vi "4x 5wire xVDTs.vi"() -> ()   [LabVIEW 2010]
uses:
  <vilib>/Platform/TimedLoop/XDataNode/XDataNode.xnode
  <vilib>/Platform/TimedLoop/XDataNode/timing_clust.ctl
  <vilib>/Platform/TimedLoop/XDataNode/nitl_modes.ctl
  <vilib>/Platform/TimedLoop/XDataNode/wakeup.ctl
  <vilib>/Platform/TimedLoop/XDataNode/XDNodeRunTimeDep.lvlib
  <vilib>/NI Veristand/FPGA/NI_VS FPGA Support.lvlib
  <userlib>/_NI VeriStand FPGA Support/NI VeriStand FPGA Clock Support/NI_VS FPGA Clock Support.lvlib
panel:
  in  "xVDT3.ScaleFactor1":i32
  in  "xVDT2.ScaleFactor2":i32
  in  "xVDT1.ScaleFactor1":i32
  in  "xVDT3.ScaleFactor2":i32
  in  "xVDT3.Scale2":fxp<+/-,19,5>
  in  "xVDT3.Scale1":fxp<+/-,19,5>
  in  "xVDT2.ScaleFactor1":i32
  in  "xVDT2.Scale2":fxp<+/-,19,5>
  in  "xVDT2.Scale1":fxp<+/-,19,5>
  in  "xVDT1.ScaleFactor2":i32
  in  "xVDT1.Scale2":fxp<+/-,19,5>
  in  "xVDT1.Scale1":fxp<+/-,19,5>
  in  "xVDT0.ScaleFactor1":i32
  in  "xVDT0.ScaleFactor2":i32
  in  "xVDT0.Scale2":fxp<+/-,19,5>
  in  "xVDT0.Scale1":fxp<+/-,19,5>
  in  "Generate IRQ":bool
  in  "Use External Timing":bool
  in  "Write to  RTSI":bool
  in  "Loop Rate (usec)":u32
  in  "Start":bool
  # "5 Wire"
  # "Configuration"
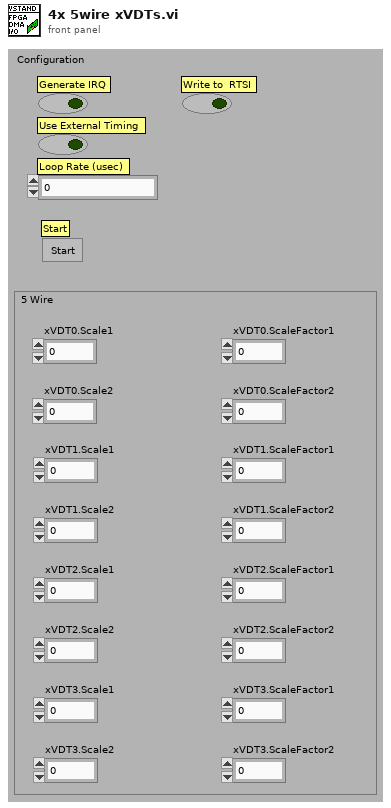
[diagram p1: front panel]
types:
  T1 = typedef "XDNodeRunTimeDep.lvlib/timing_clust.ctl" = cluster{"Expected End [f-1]":u64, "Actual End [f-1]":u64, "Finished Late? [f-1]":bool, "Expected End [i-1]":u64, "Actual End [i-1]":u64, "Finished Late? [i-1]":bool, "Expected Start [i]":u64, "Actual Start [i]":u64, "Expected Start [f]":u64, "Actual Start [f]":u64, "Source Name":string, "Structure Name":string, "Period":i64, "Deadline":i64, "Offset":i64, "Start":i64, "Priority":i32, "Timeout":i32, "Mode":T2, "Wakeup Reason":T3, "Error":errorcluster, "Source Type":string, "Secondary Source Type":string, "Global End Time":u64, "Global Start Time":u64, "Frame Duration":u64, "Iteration Duration":u64, "Assigned CPU":i32, "I/O Scan Engine Mode":u32}
  T2 = typedef "XDNodeRunTimeDep.lvlib/nitl_modes.ctl" = enum32{"No Change", "Process missed periods, maintain original phase", "Discard missed periods, maintain original phase", "Process missed periods, ignore original phase", "Discard missed periods, ignore original phase"}
  T3 = typedef "XDNodeRunTimeDep.lvlib/wakeup.ctl" = enum32{"Normal", "Aborted", "Asynchronous wakeup", "Timing source error", "Timed loop error", "Timeout"}
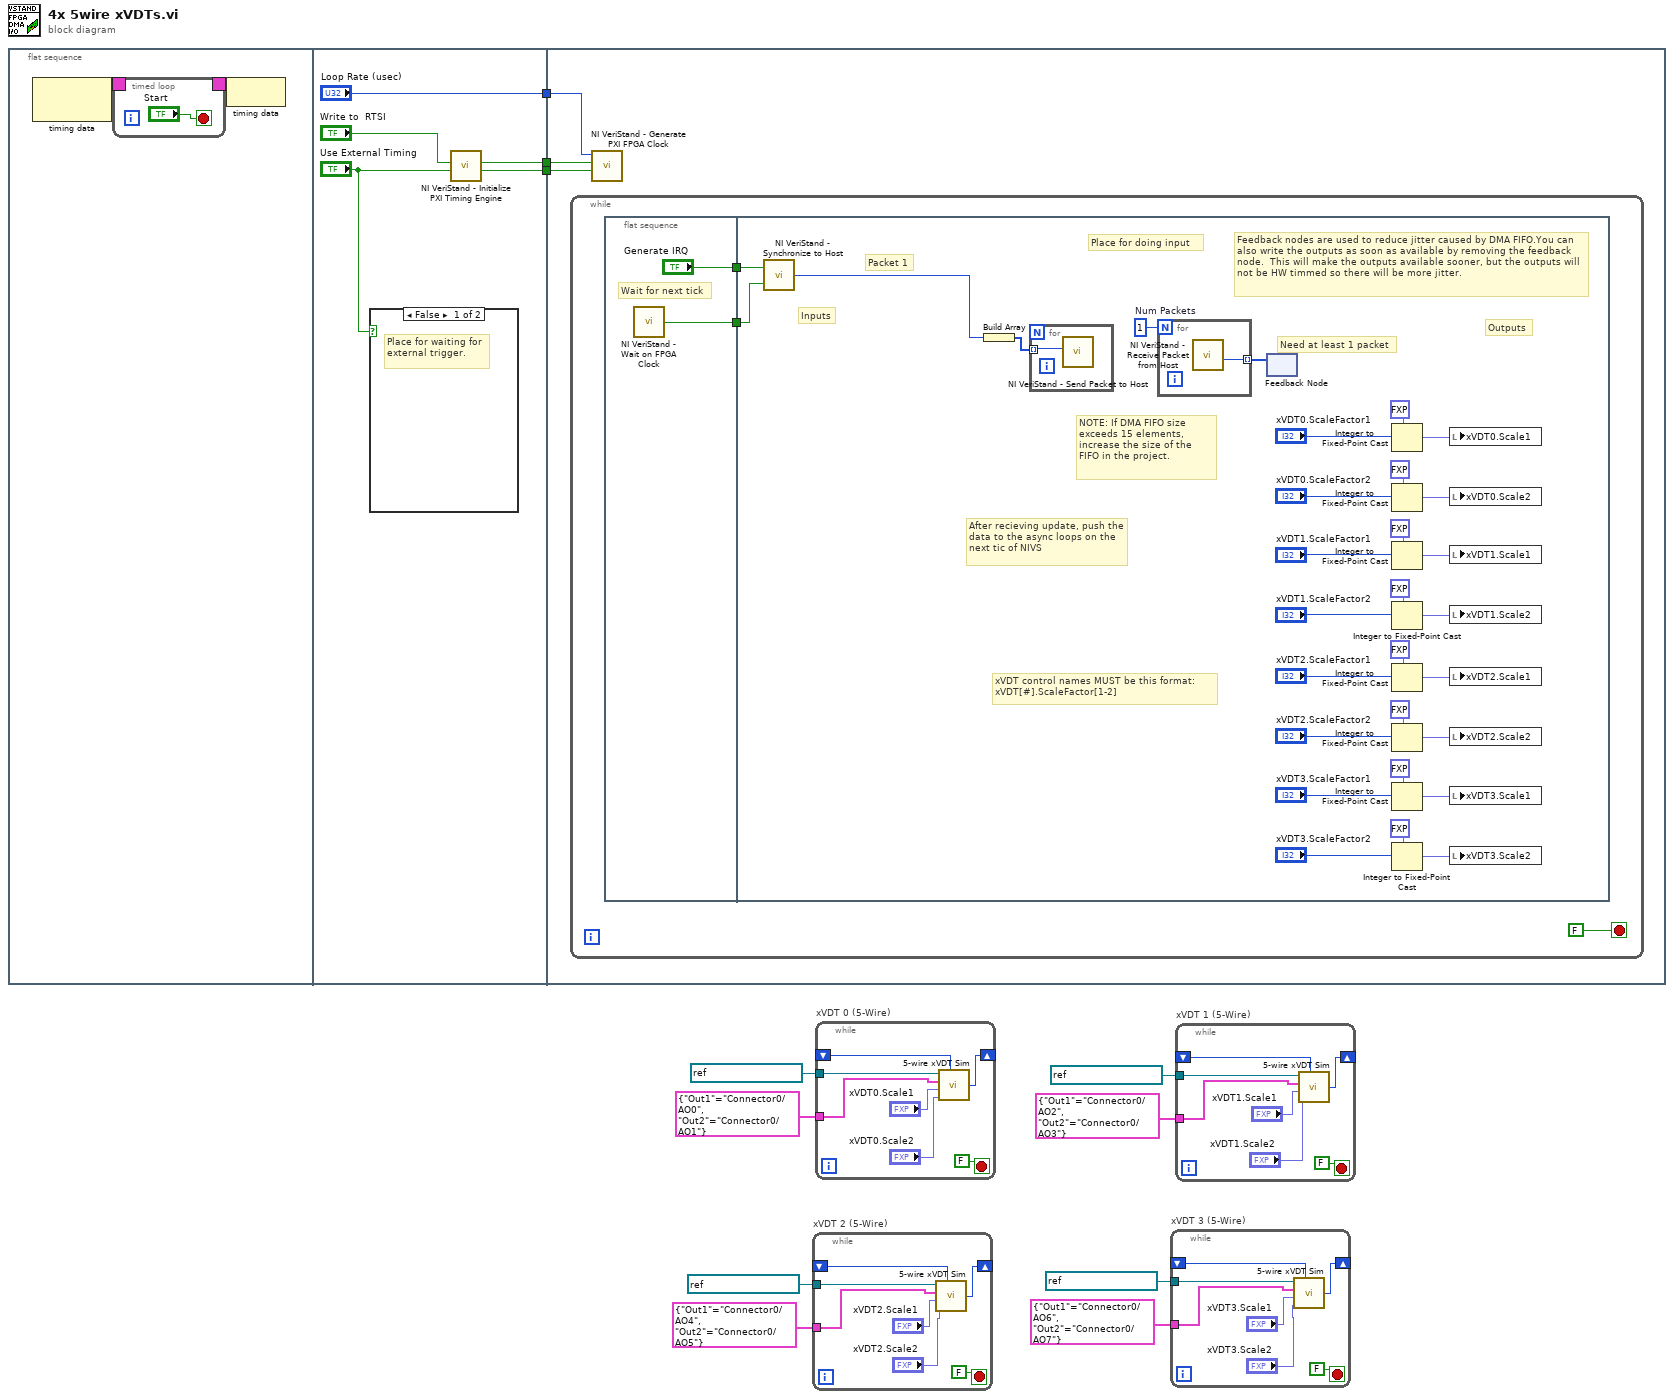
[diagram p0: block diagram]
diagram:
  n1 = flat-sequence {
    tunnel: [w20] -> w11
    tunnel: ["Loop Rate (usec)"] -> w10
    tunnel: [w19] -> w9
    tunnel: w11 -> [w26]
    tunnel: w10 -> [w25]
    tunnel: w9 -> [w24]
    frame #0 {
      n2 = node-c288() -> (w13:T1)  [unwired: 1 out]
      n3 = timed-loop {
        timing: w13 -> [_]
        timing-out: [_] -> w12
        stop <- "Start" stop-if-true
      }
      n4 = node-c288(w12) -> ()
    }
    frame #1 {
      n5 = case shown="False" "Use External Timing" {
        frame False {
          # "Place for waiting for external trigger."
        }
        frame True {
          # "Do not wait on trigger when externally timed."
        }
      }
      n6 = call <userlib>:"NI VeriStand - Initialize PXI Timing Engine.vi"("Use External Timing In"="Use External Timing", "Write to  RTSI In"="Write to  RTSI") -> ("Use External Timing Out"=w20:bool, "Write to  RTSI Out"=w19:bool)  [unwired: 8 in]
    }
    frame #2 {
      n7 = while {
        stop <- FALSE stop-if-true
        n8 = flat-sequence {
          tunnel: ["Generate IRQ"] -> w28
          tunnel: [w30] -> w27
          tunnel: w28 -> [w61]
          tunnel: w27 -> [w60]
          frame #0 {
            # "Wait for next tick"
            n9 = call <userlib>:"NI VeriStand - Wait on FPGA Clock.vi"() -> ("Clock Ticked"=w30:bool)
          }
          frame #1 {
            w57 = 1  # Num Packets
            # "xVDT control names MUST be this format:\nxVDT[#].ScaleFactor[1-2]"
            # "After recieving update, push the data to the async loops on the next tic of NIVS"
            # "Need at least 1 packet"
            # "Packet 1"
            # "Inputs"
            # "Outputs"
            # "NOTE: If DMA FIFO size exceeds 15 elements, increase the size of the FIFO in the project."
            # "Feedback nodes are used to reduce jitter caused by DMA FIFO.You can also write the outputs as soon as available by removing the feedback node.  This will make the outputs available sooner, but the outputs will not be HW timmed so there will be more jitter."
            # "Place for doing input"
            n10 = call <userlib>:"NI VeriStand - Synchronize to Host.vi"("Clock Ticked"=w60, "Generate IRQ"=w61) -> ("Is Late?"=w59:u64)
            n11 = Build Array(w59) -> (w58:u64[])
            n12 = for {
              tunnel: w58 -> [w63] mode=indexing
              n13 = call <vilib>:"NI VeriStand - Send Packet to Host.vi"("Element"=w63) -> ()  [unwired: 2 in, 9 out]
            }
            n14 = for {
              N: w57 -> [_]
              tunnel: [w62] -> w56 mode=indexing
              n15 = call <vilib>:"NI VeriStand - Receive Packet from Host.vi"() -> ("Element"=w62:u64)  [unwired: 2 in, 9 out]
            }
            n16 = feedback #1() -> ()  [unwired: 2 in]
            n17 = feedback-in #1(w56) -> ()
            n18 = Integer to Fixed-Point Cast(fixed-point type=fxp<+/-,19,5> 0.0, integer="xVDT0.ScaleFactor1") -> (fixed-point=w49:fxp<+/-,19,5>)
            n19 = Integer to Fixed-Point Cast(fixed-point type=fxp<+/-,19,5> 0.0, integer="xVDT0.ScaleFactor2") -> (fixed-point=w50:fxp<+/-,19,5>)
            n20 = Integer to Fixed-Point Cast(fixed-point type=fxp<+/-,19,5> 0.0, integer="xVDT1.ScaleFactor1") -> (fixed-point=w44:fxp<+/-,19,5>)
            n21 = Integer to Fixed-Point Cast(fixed-point type=fxp<+/-,19,5> 0.0, integer="xVDT1.ScaleFactor2") -> (fixed-point=w43:fxp<+/-,19,5>)
            n22 = Integer to Fixed-Point Cast(fixed-point type=fxp<+/-,19,5> 0.0, integer="xVDT2.ScaleFactor1") -> (fixed-point=w54:fxp<+/-,19,5>)
            n23 = Integer to Fixed-Point Cast(fixed-point type=fxp<+/-,19,5> 0.0, integer="xVDT2.ScaleFactor2") -> (fixed-point=w53:fxp<+/-,19,5>)
            n24 = Integer to Fixed-Point Cast(fixed-point type=fxp<+/-,19,5> 0.0, integer="xVDT3.ScaleFactor1") -> (fixed-point=w37:fxp<+/-,19,5>)
            n25 = Integer to Fixed-Point Cast(fixed-point type=fxp<+/-,19,5> 0.0, integer="xVDT3.ScaleFactor2") -> (fixed-point=w38:fxp<+/-,19,5>)
            n26 = local write "xVDT0.Scale1"(w49) -> ()
            n27 = local write "xVDT0.Scale2"(w50) -> ()
            n28 = local write "xVDT1.Scale1"(w44) -> ()
            n29 = local write "xVDT1.Scale2"(w43) -> ()
            n30 = local write "xVDT2.Scale1"(w54) -> ()
            n31 = local write "xVDT2.Scale2"(w53) -> ()
            n32 = local write "xVDT3.Scale1"(w37) -> ()
            n33 = local write "xVDT3.Scale2"(w38) -> ()
          }
        }
      }
      n34 = call <userlib>:"NI VeriStand - Generate PXI FPGA Clock.vi"("Use External Timing"=w26, "Write to  RTSI"=w24, "Loop Rate (usec)"=w25) -> ()  [unwired: 9 in]
    }
  }
  n35 = while "xVDT 2 (5-Wire)" {
    shift-right: [w69] -> _
    shift-left: _ -> [w70]
    tunnel: refnum<k21> "Connector0/AI2" ("FPGA I/O In") -> [w67]
    tunnel: cluster{"Out1":refnum<k21>, "Out2":refnum<k21>} {"Out1"="Connector0/AO4", "Out2"="Connector0/AO5"} ("Output Channels") -> [w66]
    stop <- FALSE stop-if-true
    n36 = call "5-wire xVDT Sim.vi"("Input Channel"=w67, "Output Channels"=w66, "xVDT#.Scale1"="xVDT2.Scale1", "xVDT#.Scale2"="xVDT2.Scale2", "Last Value"=w70) -> ("Next Value"=w69:i16)
  }
  n37 = while "xVDT 0 (5-Wire)" {
    shift-right: [w76] -> _
    shift-left: _ -> [w77]
    tunnel: refnum<k21> "Connector0/AI0" ("FPGA I/O In") -> [w74]
    tunnel: cluster{"Out1":refnum<k21>, "Out2":refnum<k21>} {"Out1"="Connector0/AO0", "Out2"="Connector0/AO1"} ("Output Channels") -> [w73]
    stop <- FALSE stop-if-true
    n38 = call "5-wire xVDT Sim.vi"("Input Channel"=w74, "Output Channels"=w73, "xVDT#.Scale1"="xVDT0.Scale1", "xVDT#.Scale2"="xVDT0.Scale2", "Last Value"=w77) -> ("Next Value"=w76:i16)
  }
  n39 = while "xVDT 3 (5-Wire)" {
    shift-right: [w83] -> _
    shift-left: _ -> [w84]
    tunnel: refnum<k21> "Connector0/AI3" ("FPGA I/O In") -> [w81]
    tunnel: cluster{"Out1":refnum<k21>, "Out2":refnum<k21>} {"Out1"="Connector0/AO6", "Out2"="Connector0/AO7"} ("Output Channels") -> [w80]
    stop <- FALSE stop-if-true
    n40 = call "5-wire xVDT Sim.vi"("Input Channel"=w81, "Output Channels"=w80, "xVDT#.Scale1"="xVDT3.Scale1", "xVDT#.Scale2"="xVDT3.Scale2", "Last Value"=w84) -> ("Next Value"=w83:i16)
  }
  n41 = while "xVDT 1 (5-Wire)" {
    shift-right: [w90] -> _
    shift-left: _ -> [w91]
    tunnel: refnum<k21> "Connector0/AI1" ("FPGA I/O In") -> [w88]
    tunnel: cluster{"Out1":refnum<k21>, "Out2":refnum<k21>} {"Out1"="Connector0/AO2", "Out2"="Connector0/AO3"} ("Output Channels") -> [w87]
    stop <- FALSE stop-if-true
    n42 = call "5-wire xVDT Sim.vi"("Input Channel"=w88, "Output Channels"=w87, "xVDT#.Scale1"="xVDT1.Scale1", "xVDT#.Scale2"="xVDT1.Scale2", "Last Value"=w91) -> ("Next Value"=w90:i16)
  }
